vi "Main.vi"(8 "error in (no error)":errorcluster, 11 "TemplateBase in":refnum<class "Cobolt.lvclass">) -> (0 "error out":errorcluster, 3 "component":refnum<class "Cobolt.lvclass">)   [LabVIEW 2012, in "Cobolt.lvclass"]
doc: "Main VI of the component."
uses:
  Cobolt.lvclass
  <vilib>/Distrio/Murmex/Murmex/command_enum.ctl
  laser lines.ctl
  Cobolt.lvclass/Cobolt.ctl
  <vilib>/Distrio/Murmex/InitialiseMessage/InitialiseMessage.lvclass
  <vilib>/Distrio/Murmex/ConfigureMessage/ConfigureMessage.lvclass
  <vilib>/Distrio/Murmex/GenericMessage/GenericMessage.lvclass
  <vilib>/Distrio/Murmex/TerminateMessage/TerminateMessage.lvclass
  <vilib>/Distrio/Murmex/Murmex/update_cluster.ctl
  <vilib>/Distrio/Murmex/Murmex/Set configure at initialise.vi
  <vilib>/Distrio/Murmex/Murmex/Set log reference.vi
  <vilib>/Distrio/Murmex/Murmex/Set VI reference.vi
  <vilib>/Distrio/Murmex/Murmex/Get ID.vi
  <vilib>/Distrio/Murmex/Murmex/Set write log to disk.vi
  <vilib>/Distrio/Murmex/Message/Add or replace parameter.vi
  <vilib>/Distrio/Murmex/Murmex/Murmex.lvclass
  <vilib>/Distrio/Murmex/Message/Message.lvclass
panel:
  in  "button::configure":bool
  in  "button:quit":bool
  in  "Tab Control":enum32{"Main", "Debug COM", "Debug Murmex"}(tab)
  in  "Power":dbl[unit]=0.05 min=0.0 max=0.05 step=0.001 format="%#_1f"
  in  "VISA command":string(combo)
  out "Error":bool
  out "Lock":bool
  out "Laser":bool
  out "Power":bool
  in  "button::Shutter":bool
  in  "button::clear faults":bool
  in  "button::apply":bool
  out "Laser line":T1=9 items=["405nm"=4, "445nm"=6, "491nm"=8, "515nm"=9, "561nm"=10]
  out "Read  from COM":string
  in  "button::set key switch":bool
  out "Error Message":string
  out "Operating mode":string
  out "Keyswitch":bool
  out "Autostart":bool
  out "Response OK":bool
  in  "button::restart laser":bool
  out "log":string
  in  "ID":string
  in  "Generic command":string
  in  "button:send command":bool
  in  "command":T2
  out "terminate?":bool
  # "LEDs"
  # "Parameters"
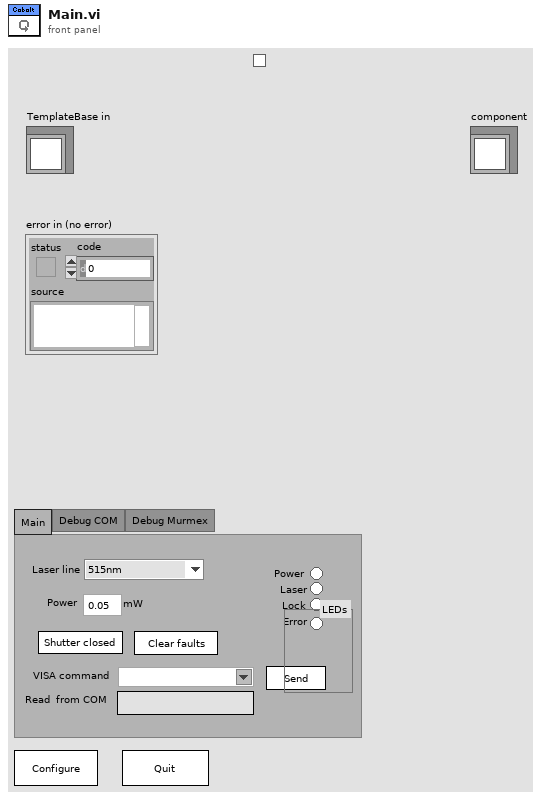
[diagram p1: front panel]
types:
  T1 = typedef "Cobolt.lvclass/laser lines.ctl" = u16
  T2 = typedef "Murmex.lvlib/Murmex.lvclass/command_enum.ctl" = enum16{"null", "initialise", "reset", "terminate", "acknowledge", "update", "inspect", "inform", "proceed", "start", "stop", "fetch", "configure", "generic"}
  T3 = enum8{"Enabled", "Disabled", "Disabled and Grayed Out"}
  T4 = typedef "Murmex.lvlib/Murmex.lvclass/update_cluster.ctl" = cluster{"target ID":string, "key chains":string[], "values":variant[]}
  T5 = typedef "Murmex.lvclass/command_enum.ctl" = enum16{"null", "initialise", "reset", "terminate", "acknowledge", "update", "inspect", "inform", "proceed", "start", "stop", "fetch", "configure", "generic"}
  T6 = typedef "Murmex.lvclass/Event type enumerations.ctl" = enum16{"before", "after"}
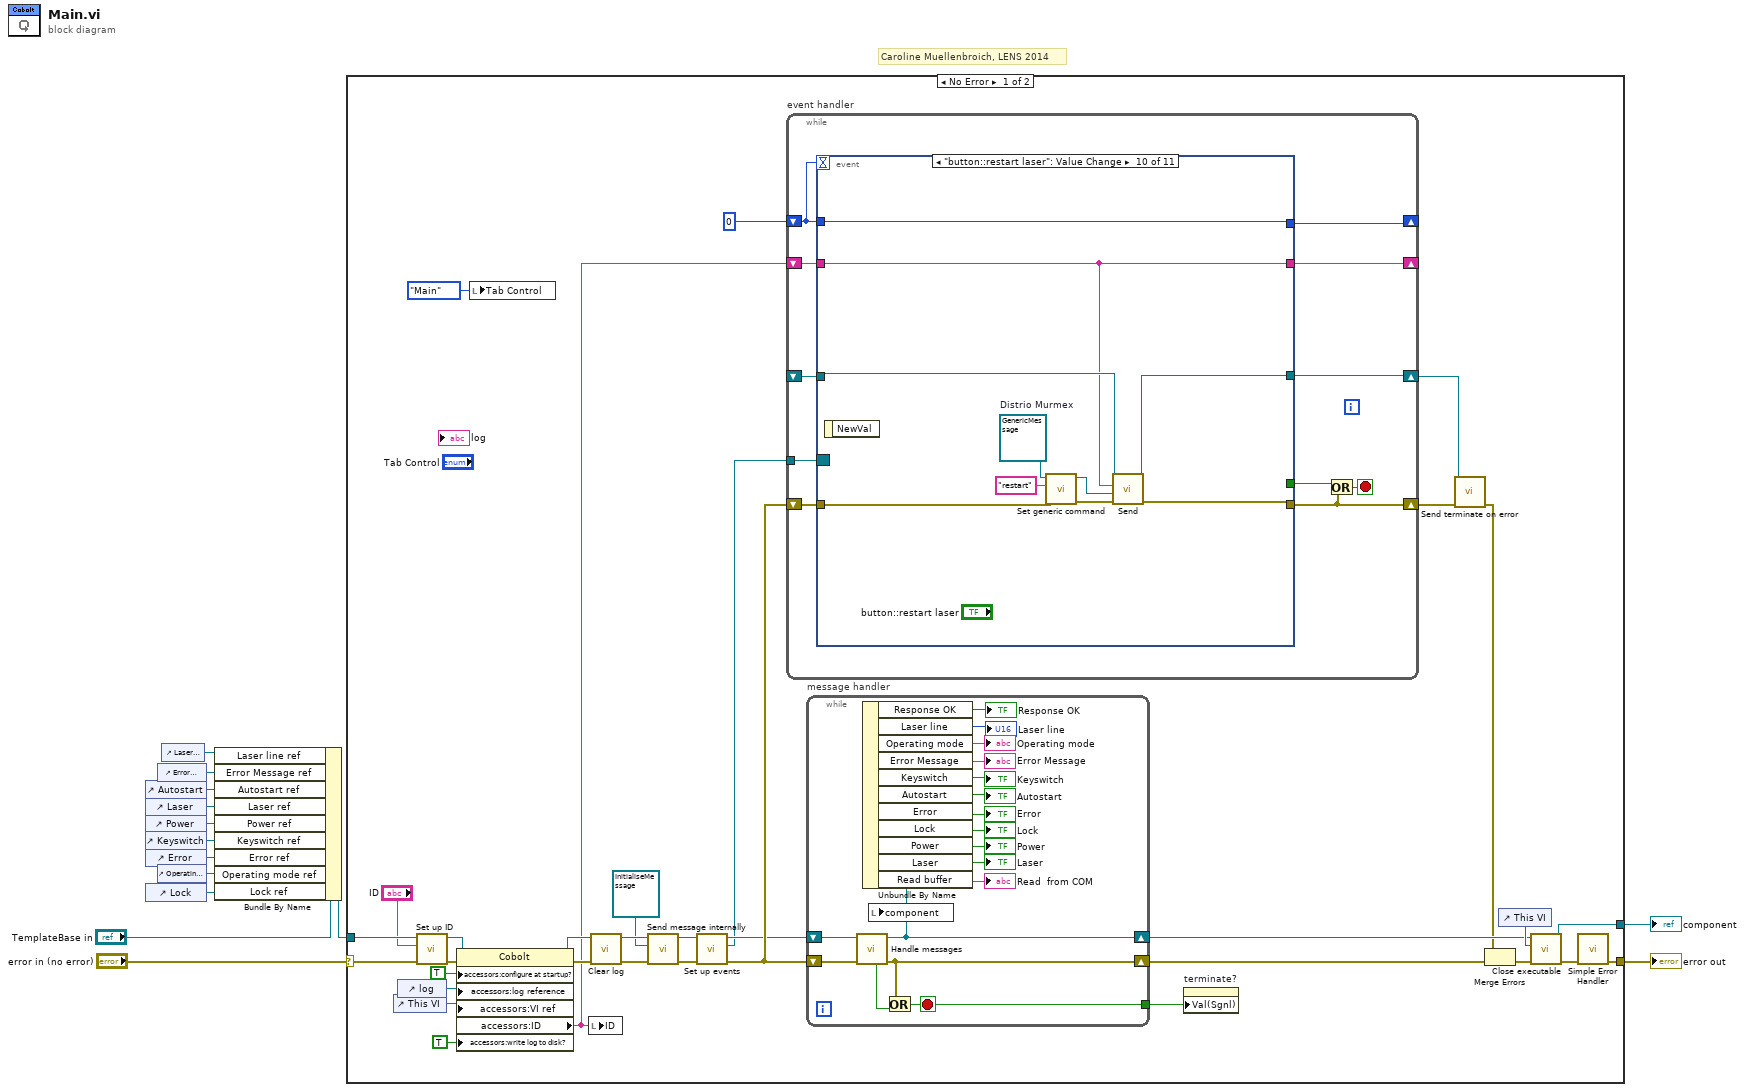
[diagram p0: block diagram]
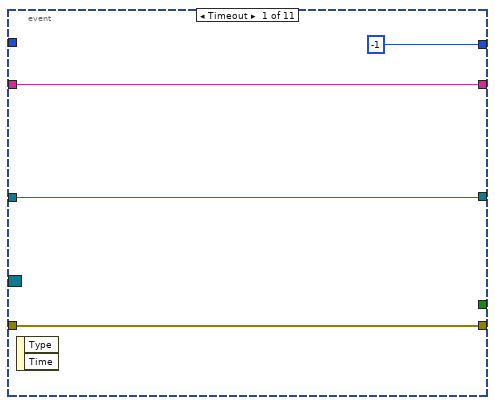
[diagram p2: hidden frame]
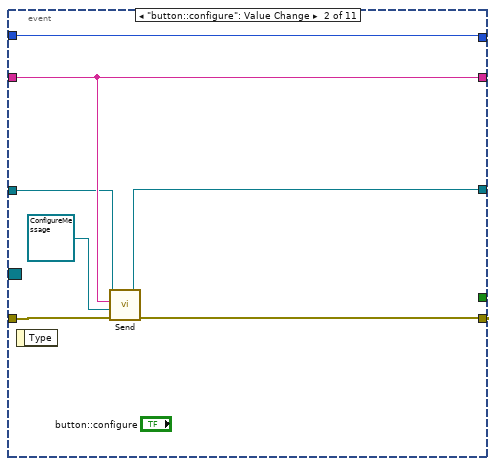
[diagram p3: hidden frame]
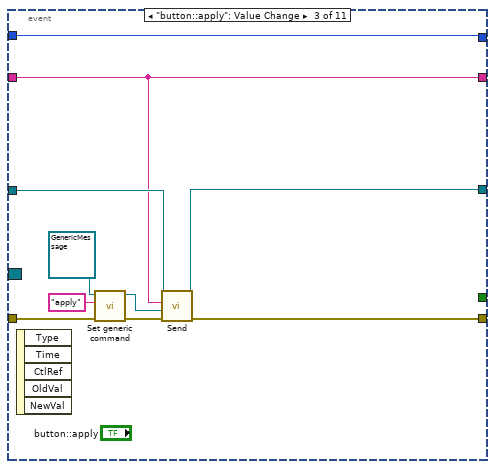
[diagram p4: hidden frame]
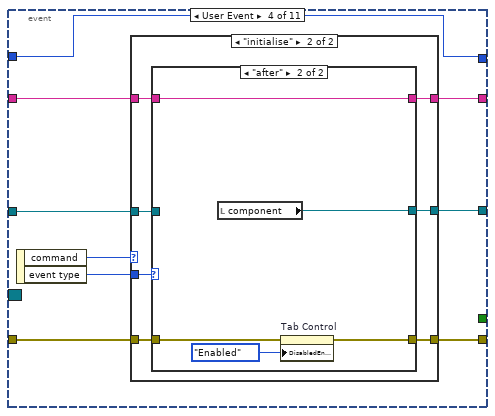
[diagram p5: hidden frame]
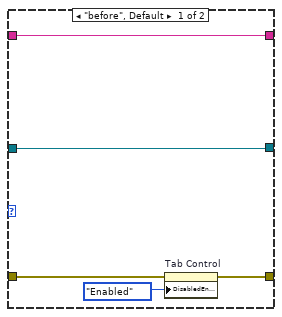
[diagram p7: hidden frame]
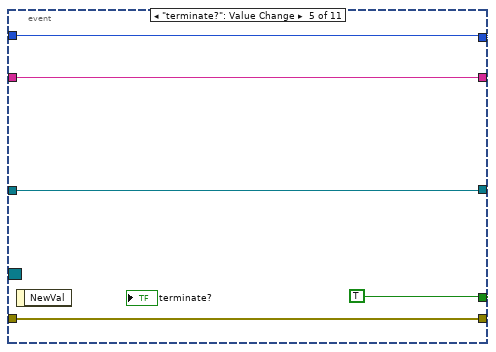
[diagram p8: hidden frame]
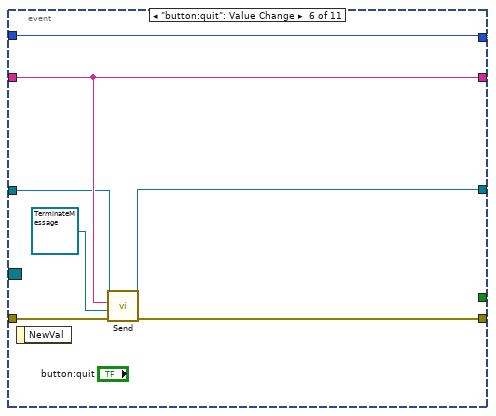
[diagram p9: hidden frame]
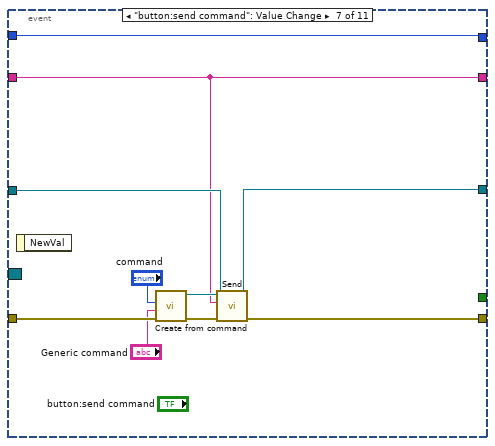
[diagram p10: hidden frame]
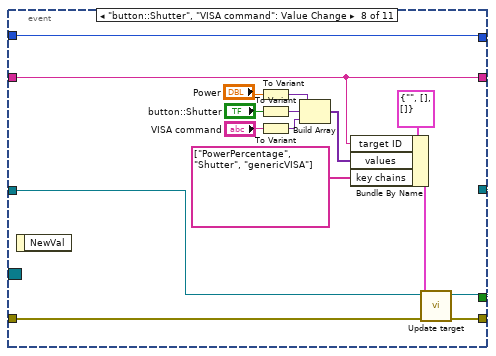
[diagram p11: hidden frame]
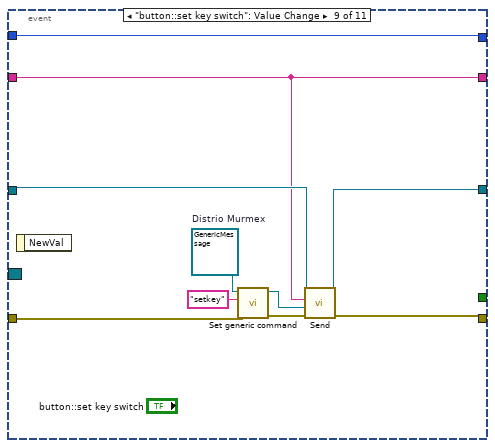
[diagram p12: hidden frame]
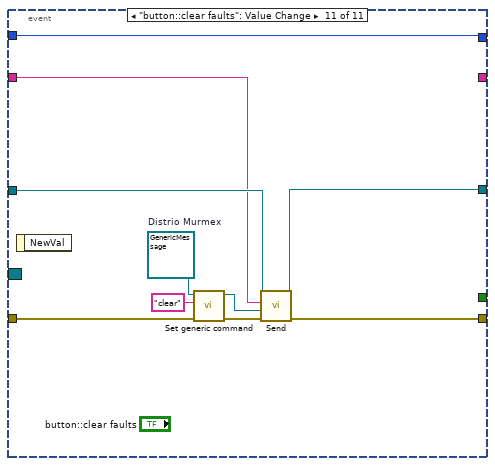
[diagram p13: hidden frame]
diagram:
  # "Caroline Muellenbroich, LENS 2014"
  n1 = control-ref of="Autostart"() -> (w3:refnum<vi>)
  n2 = control-ref of="Laser"() -> (w4:refnum<vi>)
  n3 = control-ref of="Power"() -> (w5:refnum<vi>)
  n4 = control-ref of="Keyswitch"() -> (w6:refnum<vi>)
  n5 = control-ref of="Error"() -> (w7:refnum<vi>)
  n6 = control-ref of="Lock"() -> (w9:refnum<vi>)
  n7 = control-ref of="Error Message"() -> (w2:refnum<vi>)
  n8 = control-ref of="Operating mode"() -> (w8:refnum<vi>)
  n9 = control-ref of="Laser line"() -> (w1:refnum<vi>)
  n10 = Bundle By Name(cluster="TemplateBase in", "Laser line ref"=w1, "Error Message ref"=w2, "Autostart ref"=w3, "Laser ref"=w4, "Power ref"=w5, "Keyswitch ref"=w6, "Error ref"=w7, "Operating mode ref"=w8, "Lock ref"=w9) -> (w10:refnum<class "Cobolt.lvclass">)
  n11 = case shown="No Error" "error in (no error)" {
    selector: "error in (no error)" -> [w35 w194]
    tunnel: [w28 w195] -> w14
    tunnel: w10 -> [w37 w195]
    tunnel: [w30 w194] -> w13
    frame No Error {
      n12 = control-ref of="This VI"() -> (w44:refnum<vi>)
      n13 = control-ref of="log"() -> (w45:refnum<vi>)
      n14 = call <vilib>:"Set up ID.vi"("error in (no error)"=w35, "component ID"="ID", "MurmexBase in"=w37) -> ("error out"=w38:errorcluster, "MurmexBase out"=w36:refnum<class "Cobolt.lvclass">)  [unwired: 6 in, 1 out]
      n15 = property class="Cobolt"(reference=w36, error in=w38, "accessors:configure at startup?"=TRUE ("configure at startup?"), "accessors:log reference"=w45, "accessors:VI ref"=w44, "accessors:write log to disk?"=TRUE ("write log to disk?")) -> (reference out=w47:refnum<class "Cobolt.lvclass">, error out=w42:errorcluster, "accessors:ID"=w17:string)
      n16 = local write "Tab Control"(enum32{"Main", "Debug COM", "Debug Murmex"}."Main" ("Tab Control")) -> ()
      n17 = local write "ID"(w17) -> ()
      n18 = call <vilib>:"Clear log.vi"("error in (no error)"=w42, "MurmexBase in"=w47) -> ("error out"=w41:errorcluster, "MurmexBase out"=w43:refnum<class "Cobolt.lvclass">)  [unwired: 8 in]
      n19 = call <vilib>:"Send message internally.vi"("error in (no error)"=w41, "Message"=refnum<class "InitialiseMessage.lvclass"> refnum, "Murmex in"=w43) -> ("error out"=w39:errorcluster, "Murmex out"=w27:refnum<class "Cobolt.lvclass">)  [unwired: 7 in]
      n20 = call <vilib>:"Set up events.vi"("error in (no error)"=w39, "MurmexBase in"=w27) -> ("error out"=w34:errorcluster, "Event Registration Refnum"=w22:refnum<event-registration>, "MurmexBase out"=w26:refnum<class "Cobolt.lvclass">)  [unwired: 7 in]
      n21 = while "event handler" {
        shift-right: [w57] -> w24
        shift-left: w34 -> [w58]
        shift-right: [w54] -> _
        shift-left: 0 -> [w48]
        tunnel: w22 -> [w53]
        shift-right: [w51] -> _
        shift-left: w17 -> [w52]
        shift-right: [w50] -> w20
        shift-left: _ -> [w49]
        stop <- w55 stop-if-true
        n22 = event shown="[9] \"button::restart laser\": Value Change" {
          selector: w53 -> [_ _ _ _ _ _ _ _ _ _ _]
          dyn-events: _ -> [_ _ _ _ _ _ _ _ _ _ _]
          timeout: w48 -> [_ _ _ _ _ _ _ _ _ _ _]
          tunnel: w58 -> [w62 w69 w76 w88 w113 w119 w130 w139 w152 w162 w172]
          tunnel: [w62 w64 w75 w80 w113 w120 w128 w137 w151 w161 w171] -> w57
          tunnel: [_ _ _ _ TRUE _ _ _ _ _ _] -> w56
          tunnel: w48 -> [_ w65 w71 w81 w111 w115 w122 w134 w148 w158 w167]
          tunnel: [-1 w65 w71 w81 w111 w115 w122 w134 w148 w158 w167] -> w54
          tunnel: w52 -> [w60 w68 w72 w83 w110 w118 w123 w138 w147 w157 w168]
          tunnel: [w60 w68 w72 w82 w110 w118 w123 w138 w147 w157 _] -> w51
          tunnel: [w59 w66 w73 w85 w109 w116 w125 w135 w149 w159 w169] -> w50
          tunnel: w49 -> [w59 w67 w74 w84 w109 w117 w126 w136 w150 w160 w170]
          event Timeout {
            n23 = event-data() -> ()  [unwired: 1 in, 2 out]
          }
          event "button::configure": Value Change {
            n24 = event-data() -> ()  [unwired: 1 in, 1 out]
            n25 = call <vilib>:"Send.vi"("error in (no error)"=w69, "Message"=refnum<class "ConfigureMessage.lvclass"> refnum ("Distrio Murmex"), "recipient"=w68, "Murmex in"=w67) -> ("error out"=w64:errorcluster, "Murmex out"=w66:refnum<class "Murmex.lvclass">)  [unwired: 6 in]
          }
          event "button::apply": Value Change {
            n26 = event-data() -> ()  [unwired: 1 in, 5 out]
            n27 = call <vilib>:"Set generic command.vi"("error in (no error)"=w76, "generic command"="apply", "GenericMessage in"=refnum<class "GenericMessage.lvclass"> refnum ("Distrio Murmex")) -> ("error out"=w78:errorcluster, "GenericMessage out"=w77:refnum<class "GenericMessage.lvclass">)  [unwired: 7 in]
            n28 = call <vilib>:"Send.vi"("error in (no error)"=w78, "Message"=w77, "recipient"=w72, "Murmex in"=w74) -> ("error out"=w75:errorcluster, "Murmex out"=w73:refnum<class "Murmex.lvclass">)  [unwired: 6 in]
          }
          event User Event {
            n29 = event-data() -> ("command"=w87:T5, "event type"=w86:T6)  [unwired: 1 in]
            n30 = case shown="\"initialise\"" w87 {
              tunnel: w86 -> [_ w98]
              tunnel: w88 -> [w91 w97]
              tunnel: [w91 w96] -> w80
              tunnel: [w90 w95] -> w85
              tunnel: w84 -> [w90 w94]
              tunnel: w83 -> [w89 w93]
              tunnel: [w89 w92] -> w82
              frame "null", Default {
              }
              frame "initialise" {
                n31 = case shown="\"after\"" w98 {
                  tunnel: [w102 w106] -> w96
                  tunnel: w97 -> [w103 w107]
                  tunnel: [w100 w108] -> w95
                  tunnel: w94 -> [w100 _]
                  tunnel: w93 -> [w99 w104]
                  tunnel: [w99 w104] -> w92
                  frame "before", Default {
                    n32 = property on="Tab Control" class="TabCtl (strict)"(error in=w103, "DisabledEnum"=T3."Enabled" ("Disabled")) -> (error out=w102:errorcluster)  [unwired: 1 in, 1 out]
                  }
                  frame "after" {
                    n33 = local read "component"() -> (w108:refnum<class "Cobolt.lvclass">)
                    n34 = property on="Tab Control" class="TabCtl (strict)"(error in=w107, "DisabledEnum"=T3."Enabled" ("Disabled")) -> (error out=w106:errorcluster)  [unwired: 1 in, 1 out]
                  }
                }
              }
            }
          }
          event "terminate?": Value Change {
            n35 = event-data() -> ()  [unwired: 1 in, 1 out]
          }
          event "button:quit": Value Change {
            n36 = event-data() -> ()  [unwired: 1 in, 1 out]
            n37 = call <vilib>:"Send.vi"("error in (no error)"=w119, "Message"=refnum<class "TerminateMessage.lvclass"> refnum ("Distrio Murmex 1.1:TerminateMessage"), "recipient"=w118, "Murmex in"=w117) -> ("error out"=w120:errorcluster, "Murmex out"=w116:refnum<class "Murmex.lvclass">)  [unwired: 6 in]
          }
          event "button:send command": Value Change {
            n38 = event-data() -> ()  [unwired: 1 in, 1 out]
            n39 = call <vilib>:"Create from command.vi"("error in (no error)"=w130, "generic command"="Generic command", "command"="command") -> ("error out"=w124:errorcluster, "Message out"=w129:refnum<class "Message.lvclass">)  [unwired: 7 in]
            n40 = call <vilib>:"Send.vi"("error in (no error)"=w124, "Message"=w129, "recipient"=w123, "Murmex in"=w126) -> ("error out"=w128:errorcluster, "Murmex out"=w125:refnum<class "Murmex.lvclass">)  [unwired: 6 in]
          }
          event "button::Shutter", "VISA command": Value Change {
            n41 = event-data() -> ()  [unwired: 1 in, 1 out]
            n42 = To Variant(anything="Power") -> (Variant=w146:variant)
            n43 = To Variant(anything="button::Shutter") -> (Variant=w145:variant)
            n44 = To Variant(anything="VISA command") -> (Variant=w133:variant)
            n45 = Build Array(w146, w145, w133) -> (w143:variant[])
            n46 = Bundle By Name(cluster=T4 {"target ID"="", "key chains"=[], "values"=[]} ("update cluster"), "target ID"=w138, "values"=w143, "key chains"=string[] ["PowerPercentage", "Shutter", "genericVISA"]) -> (w140:T4)
            n47 = call <vilib>:"Update target.vi"("error in (no error)"=w139, "update cluster"=w140, "MurmexBase in"=w136) -> ("error out"=w137:errorcluster, "MurmexBase out"=w135:refnum<class "Murmex.lvclass">)  [unwired: 7 in]
          }
          event "button::set key switch": Value Change {
            w156 = refnum<class "GenericMessage.lvclass"> refnum  # Distrio Murmex
            n48 = event-data() -> ()  [unwired: 1 in, 1 out]
            n49 = call <vilib>:"Set generic command.vi"("error in (no error)"=w152, "generic command"="setkey", "GenericMessage in"=w156) -> ("error out"=w154:errorcluster, "GenericMessage out"=w155:refnum<class "GenericMessage.lvclass">)  [unwired: 7 in]
            n50 = call <vilib>:"Send.vi"("error in (no error)"=w154, "Message"=w155, "recipient"=w147, "Murmex in"=w150) -> ("error out"=w151:errorcluster, "Murmex out"=w149:refnum<class "Murmex.lvclass">)  [unwired: 6 in]
          }
          event "button::restart laser": Value Change {
            w166 = refnum<class "GenericMessage.lvclass"> refnum  # Distrio Murmex
            n51 = event-data() -> ()  [unwired: 1 in, 1 out]
            n52 = call <vilib>:"Set generic command.vi"("error in (no error)"=w162, "generic command"="restart", "GenericMessage in"=w166) -> ("error out"=w164:errorcluster, "GenericMessage out"=w165:refnum<class "GenericMessage.lvclass">)  [unwired: 7 in]
            n53 = call <vilib>:"Send.vi"("error in (no error)"=w164, "Message"=w165, "recipient"=w157, "Murmex in"=w160) -> ("error out"=w161:errorcluster, "Murmex out"=w159:refnum<class "Murmex.lvclass">)  [unwired: 6 in]
          }
          event "button::clear faults": Value Change {
            w173 = refnum<class "GenericMessage.lvclass"> refnum  # Distrio Murmex
            n54 = event-data() -> ()  [unwired: 1 in, 1 out]
            n55 = call <vilib>:"Set generic command.vi"("error in (no error)"=w172, "generic command"="clear", "GenericMessage in"=w173) -> ("error out"=w175:errorcluster, "GenericMessage out"=w174:refnum<class "GenericMessage.lvclass">)  [unwired: 7 in]
            n56 = call <vilib>:"Send.vi"("error in (no error)"=w175, "Message"=w174, "recipient"=w168, "Murmex in"=w170) -> ("error out"=w171:errorcluster, "Murmex out"=w169:refnum<class "Murmex.lvclass">)  [unwired: 6 in]
          }
        }
        n57 = Or(x=w56, y=w57) -> (x .or. y?=w55:bool)
      }
      n58 = while "message handler" {
        shift-right: [w180] -> w16
        shift-left: w34 -> [w193]
        shift-right: [w179] -> w29
        shift-left: w26 -> [w192]
        tunnel: [w190] -> w40
        stop <- w190 stop-if-true
        n59 = call <vilib>:"Handle messages.vi"("error in (no error)"=w193, "Murmex in"=w192) -> ("error out"=w180:errorcluster, "Murmex out"=w179:refnum<class "Cobolt.lvclass">, "terminated?"=w191:bool)  [unwired: 7 in]
        n60 = Unbundle By Name(w179) -> ("Response OK"=→"Response OK":bool, "Laser line"=→"Laser line":T1, "Operating mode"=→"Operating mode":string, "Error Message"=→"Error Message":string, "Keyswitch"=→"Keyswitch":bool, "Autostart"=→"Autostart":bool, "Error"=→"Error":bool, "Lock"=→"Lock":bool, "Power"=→"Power":bool, "Laser"=→"Laser":bool, "Read buffer"=→"Read  from COM":string)
        n61 = local write "component"(w179) -> ()
        n62 = Or(x=w180, y=w191) -> (x .or. y?=w190:bool)
      }
      n63 = property on="terminate?" class="Bool (strict)"("Val(Sgnl)"=w40) -> ()  [unwired: 2 in, 2 out]
      n64 = call <vilib>:"Send terminate on error.vi"("error in (no error)"=w24, "Murmex in"=w20) -> ("error out"=w25:errorcluster)  [unwired: 8 in, 1 out]
      n65 = Merge Errors(w25, w16) -> (w33:errorcluster)
      n66 = control-ref of="This VI"() -> (w31:refnum<vi>)
      n67 = call <vilib>:"Close executable.vi"("error in (no error)"=w33, "main VI ref (optional)"=w31, "MurmexBase in"=w29) -> ("error out"=w32:errorcluster, "MurmexBase out"=w28:refnum<class "Cobolt.lvclass">)  [unwired: 7 in]
      n68 = call <vilib>:"Simple Error Handler.vi"("error in (no error)"=w32) -> ("error out"=w30:errorcluster)  [unwired: 4 in, 4 out]
    }
    frame Error {
    }
  }
  "error out" <- w13
  "component" <- w14
